vi "OCTavion_ScanControl_FPGA.vi"() -> ()   [LabVIEW 2016]
uses:
  <vilib>/Platform/TimedLoop/XDataNode/timing_clust.ctl
  <vilib>/Platform/TimedLoop/XDataNode/nitl_modes.ctl
  <vilib>/Platform/TimedLoop/XDataNode/wakeup.ctl
  <vilib>/rvi/Emulation/niFpgaGetClockAttributes.vi
  <vilib>/rvi/Emulation/niFpgaSctlEmulationGetInTimedLoop.vi
  <vilib>/rvi/Emulation/niFpgaEmulationReportErrorSimple.vi
  <vilib>/rvi/Emulation/niFpgaCriticalErrorInLSC.vi
  <vilib>/rvi/eio/common/nirviEmuTemplateMethod_errors.vi
  <vilib>/platform/TimedLoop/XDataNode/XDataNode.xnode
  <vilib>/eio/EIONode/EIONode.xnode
  <vilib>/Platform/TimedLoop/XDataNode/XDNodeRunTimeDep.lvlib
panel:
  in  "ScanParameters":T1
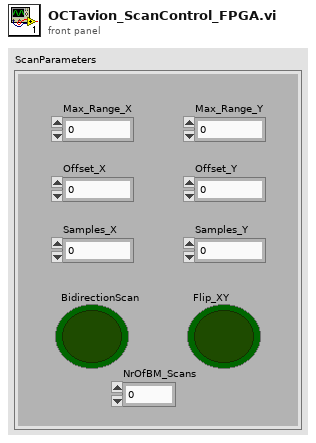
[diagram p1: front panel]
types:
  T1 = cluster{"Max_Range_X":u16, "Max_Range_Y":u16, "Offset_X":i16, "Offset_Y":i16, "Samples_X":u16, "Samples_Y":u16, "BidirectionScan":bool, "Flip_XY":bool, "NrOfBM_Scans":u16}
  T2 = typedef "XDNodeRunTimeDep.lvlib/timing_clust.ctl" = cluster{"Expected End [f-1]":u64, "Actual End [f-1]":u64, "Finished Late? [f-1]":bool, "Expected End [i-1]":u64, "Actual End [i-1]":u64, "Finished Late? [i-1]":bool, "Expected Start [i]":u64, "Actual Start [i]":u64, "Expected Start [f]":u64, "Actual Start [f]":u64, "Source Name":string, "Structure Name":string, "Period":i64, "Deadline":i64, "Offset":i64, "Start":i64, "Priority":i32, "Timeout":i32, "Mode":T3, "Wakeup Reason":T4, "Error":errorcluster, "Source Type":string, "Secondary Source Type":string, "Global End Time":u64, "Global Start Time":u64, "Frame Duration":u64, "Iteration Duration":u64, "Assigned CPU":i32, "I/O Scan Engine Mode":u32}
  T3 = typedef "XDNodeRunTimeDep.lvlib/nitl_modes.ctl" = enum32{"No Change", "Process missed periods, maintain original phase", "Discard missed periods, maintain original phase", "Process missed periods, ignore original phase", "Discard missed periods, ignore original phase"}
  T4 = typedef "XDNodeRunTimeDep.lvlib/wakeup.ctl" = enum32{"Normal", "Aborted", "Asynchronous wakeup", "Timing source error", "Timed loop error", "Timeout"}
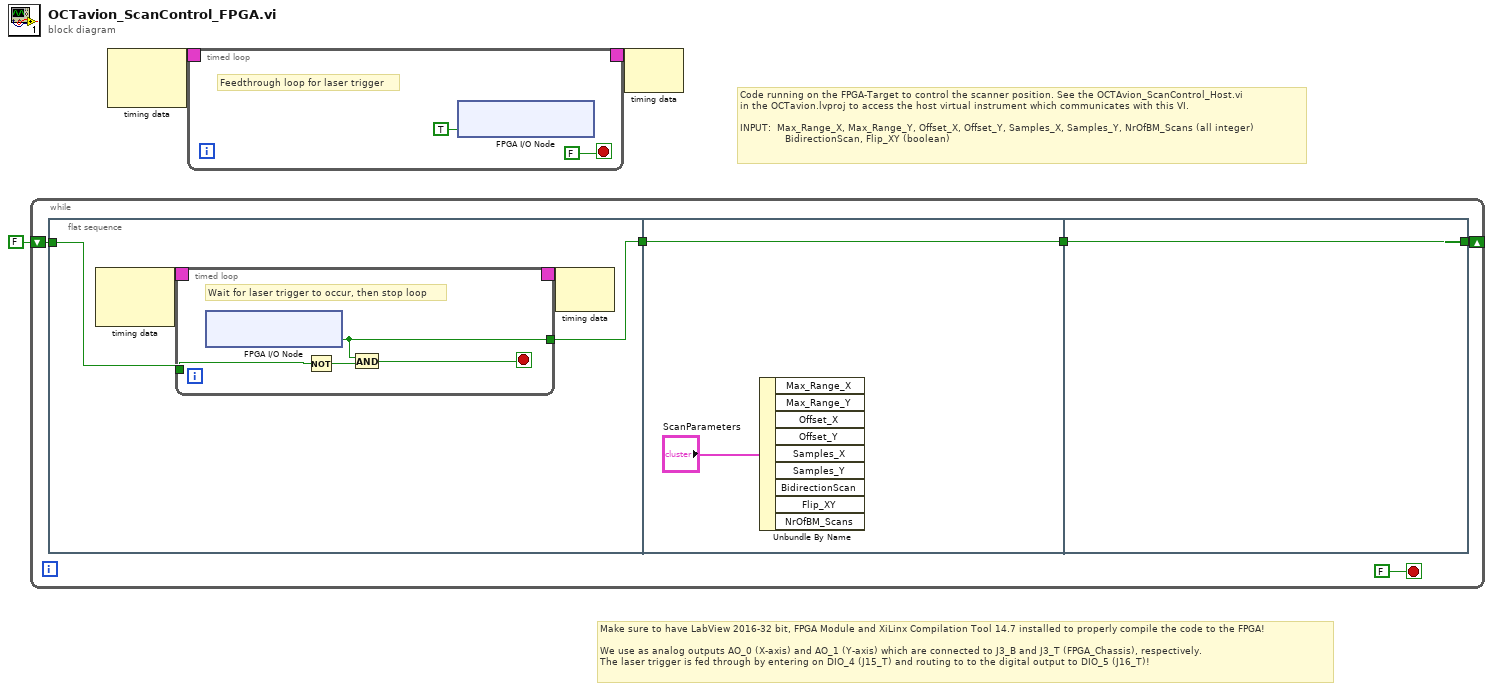
[diagram p0: block diagram]
diagram:
  # "Make sure to have LabView 2016-32 bit, FPGA Module and XiLinx Compilation Tool 14.7 installed to properly compile the code to the FPGA!\n\nWe use as analog outputs AO_0 (X-axis) and AO_1 (Y-axis) which are connected to J3_B and J3_T (FPGA_Chassis), respectively.\nThe laser trigger is fed through by entering on DIO_4 (J15_T) and routing to to the digital output to DIO_5 (J16_T)!"
  # "Code running on the FPGA-Target to control the scanner position. See the OCTAvion_ScanControl_Host.vi\nin the OCTavion.lvproj to access the host virtual instrument which communicates with this VI.\n\nINPUT:  Max_Range_X, Max_Range_Y, Offset_X, Offset_Y, Samples_X, Samples_Y, NrOfBM_Scans (all integer)\n               BidirectionScan, Flip_XY (boolean)"
  n1 = while {
    shift-right: [w7] -> _
    shift-left: FALSE ("Connector0/DIO4") -> [w4]
    stop <- FALSE stop-if-true
    n2 = flat-sequence {
      tunnel: [w10] -> w5
      tunnel: w4 -> [w9]
      tunnel: [w22] -> w6
      tunnel: w5 -> [w22]
      tunnel: [w23] -> w7
      tunnel: w6 -> [w23]
      frame #0 {
        n3 = node-c288() -> (w12:T2)  [unwired: 2 in]
        n4 = timed-loop {
          timing: w12 -> [_]
          timing-out: [_] -> w11
          tunnel: [w16] -> w10
          tunnel: w9 -> [w14]
          stop <- w13 stop-if-true
          # "Wait for laser trigger to occur, then stop loop"
          n5 = xnode "FPGA I/O Node"() -> ("Connector0/DIO6"=w16:bool)  [unwired: 1 in, 1 out]
          n6 = Not(x=w14) -> (.not. x?=w15:bool)
          n7 = And(x=w16, y=w15) -> (x .and. y?=w13:bool)
        }
        n8 = node-c288(w11) -> ()  [unwired: 1 out]
      }
      frame #1 {
        n9 = Unbundle By Name("ScanParameters") -> ()  [unwired: 9 out]
      }
      frame #2 {
      }
    }
  }
  n10 = node-c288() -> (w3:T2)  [unwired: 2 in]
  n11 = timed-loop {
    timing: w3 -> [_]
    timing-out: [_] -> w2
    stop <- FALSE stop-if-true
    # "Feedthrough loop for laser trigger"
    n12 = xnode "FPGA I/O Node"("Connector0/DIO0"=TRUE) -> ()  [unwired: 1 in, 1 out]
  }
  n13 = node-c288(w2) -> ()  [unwired: 1 out]
